vi "Find Application Type and Folder.vi"(5 "error IN":errorcluster) -> (14 "Application:Kind":T1(ring), 16 "Application Folder":path, 19 "error out":errorcluster)   [LabVIEW 2020, in "Generic Utilities.lvclass"]
uses:
  Generic Utilities.lvclass
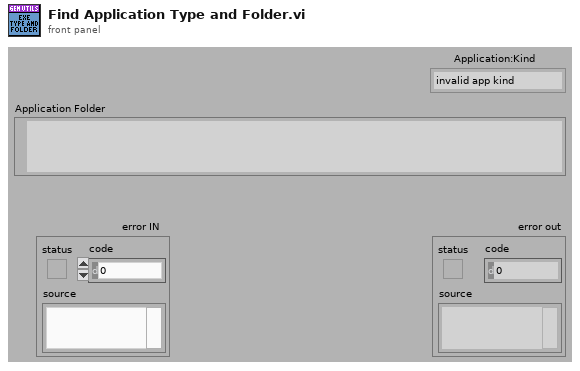
[diagram p1: front panel]
types:
  T1 = enum32{"invalid app kind", "Development System", "Run Time System", "Student Edition", "Embedded LabVIEW", "Evaluation", "Custom"}
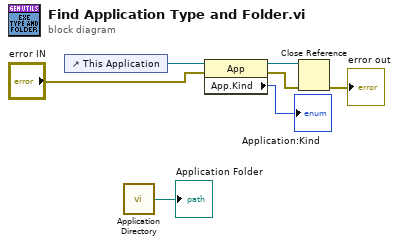
[diagram p0: block diagram]
diagram:
  n1 = control-ref of="This Application"() -> (w7:refnum<vi>)
  n2 = call <vilib>:"Application Directory.vi"() -> ("Application Directory"=→"Application Folder":path)
  n3 = property class="App"(reference=w7, error in="error IN") -> (reference out=w5:refnum<vi>, error out=w4:errorcluster, "App.Kind"=→"Application:Kind":T1)
  n4 = Close Reference(reference=w5, error in (no error)=w4) -> (error out=→"error out":errorcluster)
